vi "ztscopeM Vertical Query.vi"(0 "Instrument Handle In":i32, 5 "Channel":i32(ring) items=["Input Channel 1", "Input Channel 2", "Input Channel 3", "Input Channel 4"], 11 "error in":errorcluster) -> (3 "Attenuation":dbl, 4 "Instrument Handle Out":i32, 6 "Range":dbl, 8 "Offset":dbl, 10 "Coupling":i32, 13 "Lowpass Filter":i32, 14 "Impedance":dbl, 15 "error out":errorcluster)   [LabVIEW 2013]
doc: "Query the vertical settings for the selected channel"
uses:
  ztscopeM.dll
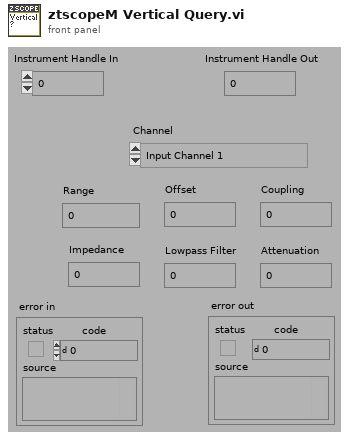
[diagram p1: front panel]
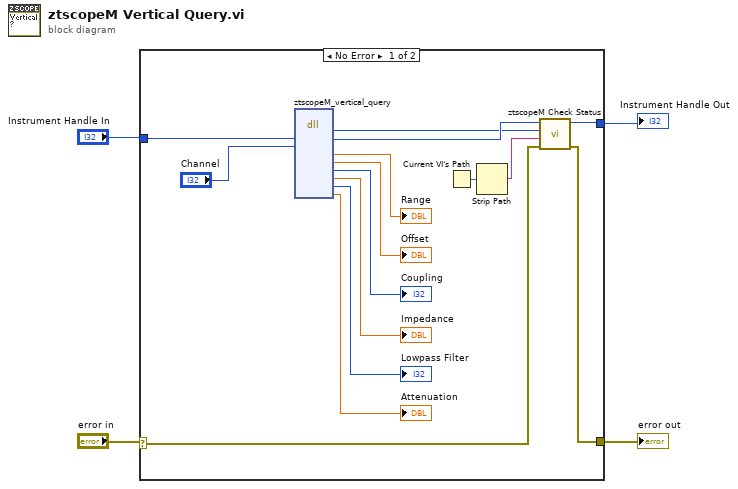
[diagram p0: block diagram]
diagram:
  n1 = case shown="No Error" "error in" {
    selector: "error in" -> [w7 w21]
    tunnel: [w6 w21] -> w1
    tunnel: "Instrument Handle In" -> [w19 w20]
    tunnel: [w5 w20] -> w3
    frame No Error {
      n2 = dll-call lib="C:/Program Files/National Instruments/instr.lib/ztscopem/ztscopeM.dll" fn="ztscopeM_vertical_query"("instrumentHandle"=w19, "channel"="Channel") -> (w8:i32, "instrumentHandle"=w9:i32, "range"=→"Range":dbl, "offset"=→"Offset":dbl, "coupling"=→"Coupling":i32, "impedance"=→"Impedance":dbl, "lowpassFilter"=→"Lowpass Filter":i32, "attenuation"=→"Attenuation":dbl)  [unwired: 10 in, 2 out]
      n3 = Current VI's Path() -> (path=w11:path)
      n4 = Strip Path(path=w11) -> (name=w10:string)  [unwired: 1 out]
      n5 = call "ztscopeM Check Status.vi"("error in"=w7, "name of VI"=w10, "status"=w8, "instrument handle in"=w9) -> ("error out"=w6:errorcluster, "instrument handle out"=w5:i32)  [unwired: 2 in]
    }
    frame Error {
    }
  }
  "Instrument Handle Out" <- w3
  "error out" <- w1
